vi "inputTypeStringToDAQmx.vi"(10 "inputConfig":T1 caption="Input\nConfig") -> (2 "input terminal configuration":i32(ring)=10106 items=["default"=-1, "RSE"=10083, "NRSE"=10078, "Differential"=10106, "Pseudodifferential"=12529])   [LabVIEW 2022 SP3]
uses:
  Controls/DAQinputType.ctl
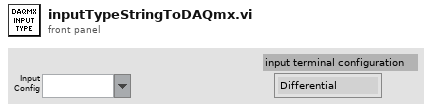
[diagram p1: front panel]
types:
  T1 = typedef "DAQinputType.ctl" = string
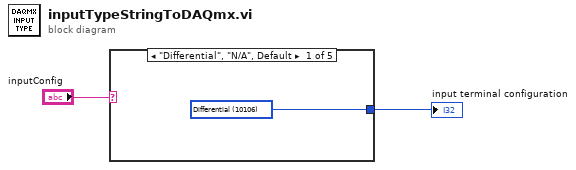
[diagram p0: block diagram]
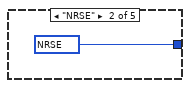
[diagram p2: hidden frame]
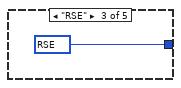
[diagram p3: hidden frame]
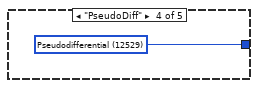
[diagram p4: hidden frame]
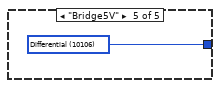
[diagram p5: hidden frame]
diagram:
  n1 = case shown="\"Differential\", \"N/A\", Default" "inputConfig" {
    tunnel: [w3 w4 w5 w6 w7] -> w1
    frame "Differential", "N/A", Default {
      w3 = 10106 items=["default"=-1, "RSE"=10083, "NRSE"=10078, "Differential"=10106, "Pseudodifferential"=12529] ("input terminal configuration")
    }
    frame "NRSE" {
      w4 = 10078 items=["default"=-1, "RSE"=10083, "NRSE"=10078, "Differential"=10106, "Pseudodifferential"=12529] ("input terminal configuration")
    }
    frame "RSE" {
      w5 = 10083 items=["default"=-1, "RSE"=10083, "NRSE"=10078, "Differential"=10106, "Pseudodifferential"=12529] ("input terminal configuration")
    }
    frame "PseudoDiff" {
      w6 = 12529 items=["default"=-1, "RSE"=10083, "NRSE"=10078, "Differential"=10106, "Pseudodifferential"=12529] ("input terminal configuration")
    }
    frame "Bridge5V" {
      w7 = 10106 items=["default"=-1, "RSE"=10083, "NRSE"=10078, "Differential"=10106, "Pseudodifferential"=12529] ("input terminal configuration")
    }
  }
  "input terminal configuration" <- w1
